vi "GetWindowFullscreenMode.vi"(8 "No Error":errorcluster, 11 "Window [SDL_Window *]":i64 format="%.0x") -> (0 "Error Out":errorcluster, 2 "Borderless Fullscreen Mode":bool, 3 "Display Mode":T1)   [LabVIEW 2026, in "SDL3.lvlib" / "Video.lvlib"]
doc: "<B>Summary</B>\nQuery the display mode to use when a window is visible at fullscreen.\n\n<B>Remarks</B>\nReturns a pointer to the exclusive fullscreen mode to use or NULL for borderless fullscreen desktop mode."
uses:
  Video.lvlib
  DisplayMode--cluster.ctl
  DisplayID--integer.ctl
  Pixels/PixelFormat--enum.ctl
  Dereference-DisplayMode.vi/333b0950-9307-44e2-9434-6a524a6d6aa0.vi
  Dereference-DisplayMode.vi/0bdeca21-8044-45ae-b16c-a9778b4cc95d.vi
  Pixels/U32ToPixelFormatEnum.vi
  Lib/SDL3.dll
  Pixels/Pixels.lvlib
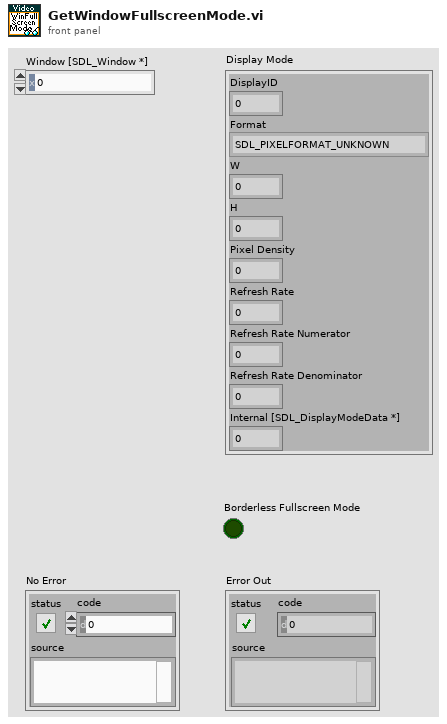
[diagram p1: front panel]
types:
  T1 = typedef "SDL3.lvlib/Video.lvlib/DisplayMode--cluster.ctl" = cluster{"DisplayID":T2, "Format":T3, "W":i32, "H":i32, "Pixel Density":sgl, "Refresh Rate":sgl, "Refresh Rate Numerator":i32, "Refresh Rate Denominator":i32, "Internal [SDL_DisplayModeData *]":i64}
  T2 = typedef "SDL3.lvlib/Video.lvlib/DisplayID--integer.ctl" = u32
  T3 = typedef "SDL3.lvlib/Pixels.lvlib/PixelFormat--enum.ctl" = enum32{"SDL_PIXELFORMAT_UNKNOWN", "SDL_PIXELFORMAT_INDEX1LSB", "SDL_PIXELFORMAT_INDEX1MSB", "SDL_PIXELFORMAT_INDEX2LSB", "SDL_PIXELFORMAT_INDEX2MSB", "SDL_PIXELFORMAT_INDEX4LSB", "SDL_PIXELFORMAT_INDEX4MSB", "SDL_PIXELFORMAT_INDEX8", "SDL_PIXELFORMAT_RGB332", "SDL_PIXELFORMAT_XRGB4444", "SDL_PIXELFORMAT_XBGR4444", "SDL_PIXELFORMAT_XRGB1555", "SDL_PIXELFORMAT_XBGR1555", "SDL_PIXELFORMAT_ARGB4444", "SDL_PIXELFORMAT_RGBA4444", "SDL_PIXELFORMAT_ABGR4444", "SDL_PIXELFORMAT_BGRA4444", "SDL_PIXELFORMAT_ARGB1555", "SDL_PIXELFORMAT_RGBA5551", "SDL_PIXELFORMAT_ABGR1555", "SDL_PIXELFORMAT_BGRA5551", "SDL_PIXELFORMAT_RGB565", "SDL_PIXELFORMAT_BGR565", "SDL_PIXELFORMAT_RGB24", "SDL_PIXELFORMAT_BGR24", "SDL_PIXELFORMAT_XRGB8888", "SDL_PIXELFORMAT_RGBX8888", "SDL_PIXELFORMAT_XBGR8888", "SDL_PIXELFORMAT_BGRX8888", "SDL_PIXELFORMAT_ARGB8888", "SDL_PIXELFORMAT_RGBA8888", "SDL_PIXELFORMAT_ABGR8888", "SDL_PIXELFORMAT_BGRA8888", "SDL_PIXELFORMAT_XRGB2101010", "SDL_PIXELFORMAT_XBGR2101010", "SDL_PIXELFORMAT_ARGB2101010", "SDL_PIXELFORMAT_ABGR2101010", "SDL_PIXELFORMAT_RGB48", "SDL_PIXELFORMAT_BGR48", "SDL_PIXELFORMAT_RGBA64", "SDL_PIXELFORMAT_ARGB64", "SDL_PIXELFORMAT_BGRA64", "SDL_PIXELFORMAT_ABGR64", "SDL_PIXELFORMAT_RGB48_FLOAT", "SDL_PIXELFORMAT_BGR48_FLOAT", "SDL_PIXELFORMAT_RGBA64_FLOAT", "SDL_PIXELFORMAT_ARGB64_FLOAT", "SDL_PIXELFORMAT_BGRA64_FLOAT", "SDL_PIXELFORMAT_ABGR64_FLOAT", "SDL_PIXELFORMAT_RGB96_FLOAT", "SDL_PIXELFORMAT_BGR96_FLOAT", "SDL_PIXELFORMAT_RGBA128_FLOAT", "SDL_PIXELFORMAT_ARGB128_FLOAT", "SDL_PIXELFORMAT_BGRA128_FLOAT", "SDL_PIXELFORMAT_ABGR128_FLOAT", "SDL_PIXELFORMAT_YV12", "SDL_PIXELFORMAT_IYUV", "SDL_PIXELFORMAT_YUY2", "SDL_PIXELFORMAT_UYVY", "SDL_PIXELFORMAT_YVYU", "SDL_PIXELFORMAT_NV12", "SDL_PIXELFORMAT_NV21", "SDL_PIXELFORMAT_P010", "SDL_PIXELFORMAT_EXTERNAL_OES"}
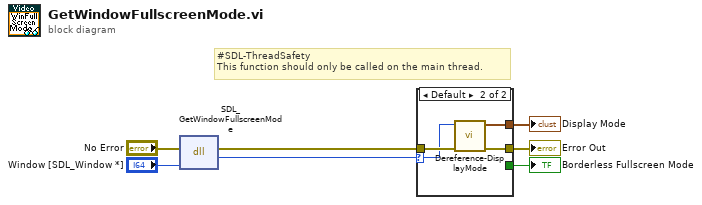
[diagram p0: block diagram]
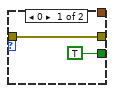
[diagram p2: hidden frame]
diagram:
  # "#SDL-ThreadSafety\nThis function should only be called on the main thread."
  n1 = dll-call lib="C:/Users/saukko/Dev/LV-SDL3/Sources/SDL3/Lib/SDL3.*" fn="SDL_GetWindowFullscreenMode"(error in="No Error", "window"="Window [SDL_Window *]") -> (error out=w5:errorcluster, "return type"=w4:i64)  [unwired: 3 in, 1 out]
  n2 = case shown="Default" w4 {
    selector: w4 -> [_ w12]
    tunnel: w5 -> [w9 w13]
    tunnel: [w9 w11] -> w3
    tunnel: [_ w10] -> w2
    tunnel: [TRUE ("Borderless Fullscreen Mode") _] -> w1
    frame 0 {
    }
    frame Default {
      n3 = call "Dereference-DisplayMode.vi"("error in (no error)"=w13, "[SDL_DisplayMode*]"=w12) -> ("error out"=w11:errorcluster, "Display Mode"=w10:T1)  [unwired: 8 in]
    }
  }
  "Error Out" <- w3
  "Display Mode" <- w2
  "Borderless Fullscreen Mode" <- w1
